vi "Create Item Name.vi"(6 "Parent":i32, 7 "Hide Full Name? (F)":bool, 10 "Type":variant, 11 "Item Graph In":T1[](array[typedef])) -> (2 "Name":string, 3 "Item Graph":T1[](array[typedef]))   [LabVIEW 2020, in "Better Search.lvlib"]
uses:
  Better Search.lvlib
  Data Types/Type Reflection Item.ctl
  <vilib>/Utility/Data Type/NI_Data Type.lvlib
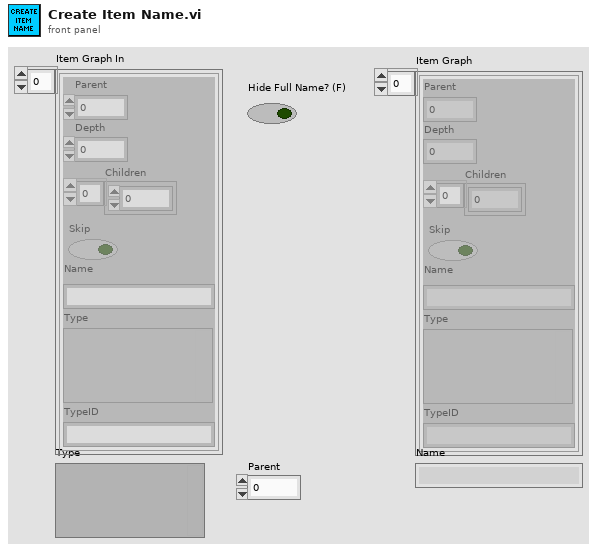
[diagram p1: front panel]
types:
  T1 = typedef "Better Search.lvlib/Type Reflection Item.ctl" = cluster{"Parent":i32, "Depth":i32, "Children":i32[], "Skip":bool, "Name":string, "Type":variant, "TypeID":string}
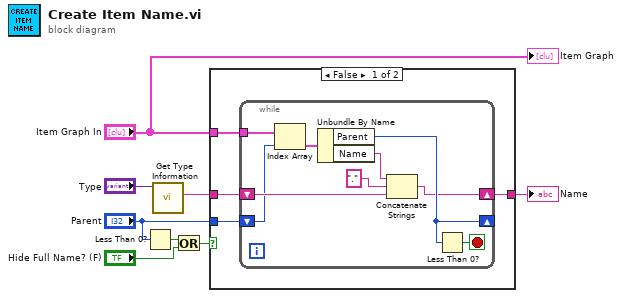
[diagram p0: block diagram]
diagram:
  n1 = Less Than 0?(x="Parent") -> (x < 0?=w5:bool)
  n2 = call <vilib>:"Get Type Information.vi"("variant"="Type") -> ("name"=w7:string)  [unwired: 6 in, 4 out]
  n3 = Or(x=w5, y="Hide Full Name? (F)") -> (x .or. y?=w3:bool)
  n4 = case shown="False" w3 {
    tunnel: w7 -> [w11 w22]
    tunnel: [w10 w22] -> w6
    tunnel: "Item Graph In" -> [w9 _]
    tunnel: "Parent" -> [w12 _]
    frame False {
      n5 = while {
        shift-right: [w18] -> _
        shift-left: w12 -> [w13]
        shift-right: [w14] -> w10
        shift-left: w11 -> [w17]
        tunnel: w9 -> [w20]
        stop <- w21 stop-if-true
        n6 = Index Array(array=w20, index=w13) -> (element=w19:T1)
        n7 = Unbundle By Name(w19) -> ("Parent"=w18:i32, "Name"=w16:string)
        n8 = Concatenate Strings(w16, "." ("string"), w17) -> (w14:string)
        n9 = Less Than 0?(x=w18) -> (x < 0?=w21:bool)
      }
    }
    frame True {
    }
  }
  "Name" <- w6
  "Item Graph" <- "Item Graph In"
